vi "createFilePath.vi"(10 "fileSuffix":string, 11 "Base Path":path=path "D:/") -> (2 "appended path":path)   [LabVIEW 2018]
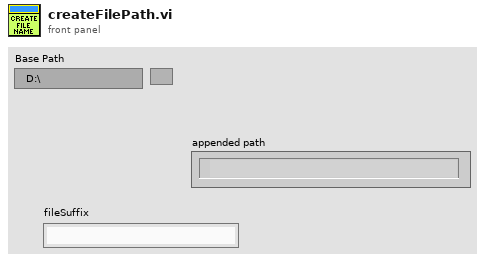
[diagram p1: front panel]
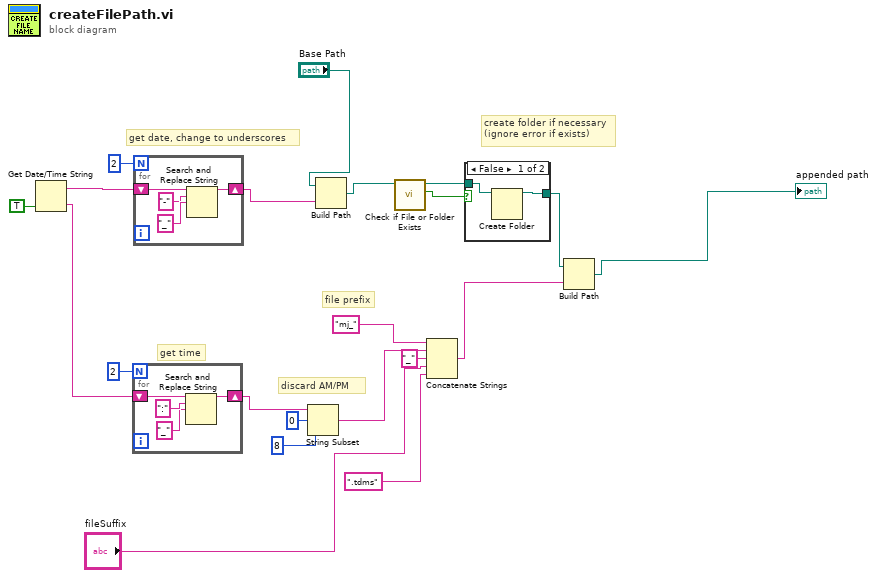
[diagram p0: block diagram]
diagram:
  # "file prefix"
  # "create folder if necessary\n(ignore error if exists)"
  # "get time"
  # "discard AM/PM"
  # "get date, change to underscores"
  n1 = Get Date/Time String(want seconds? (F)=TRUE) -> (date string=w18:string, time string=w17:string)  [unwired: 2 in]
  n2 = for {
    N: 2 -> [_]
    shift-right: [w22] -> w16
    shift-left: w17 -> [w25]
    n3 = Search and Replace String(input string=w25, search string=":", replace string="_" ("replace string (\"\")")) -> (result string=w22:string)  [unwired: 5 in, 3 out]
  }
  n4 = for {
    N: 2 -> [_]
    shift-right: [w26] -> w11
    shift-left: w18 -> [w27]
    n5 = Search and Replace String(input string=w27, search string="-", replace string="_" ("replace string (\"\")")) -> (result string=w26:string)  [unwired: 5 in, 3 out]
  }
  n6 = String Subset(string=w16, offset (0)=0, length (rest)=8 ("length (rest)")) -> (substring=w15:string)
  n7 = Build Path(base path="Base Path", name or relative path=w11) -> (appended path=w7:path)
  n8 = call <vilib>:"Check if File or Folder Exists.vi"("path"=w7) -> ("file or folder exists?"=w6:bool, "dup path"=w5:path)  [unwired: 8 in, 1 out]
  n9 = Concatenate Strings("mj_" ("string"), w15, "_" ("string"), "fileSuffix", ".tdms" ("string")) -> (w9:string)
  n10 = case shown="False" w6 {
    tunnel: [w31 w32] -> w10
    tunnel: w5 -> [w30 w32]
    frame False {
      n11 = Create Folder(path (use dialog)=w30) -> (created path=w31:path)  [unwired: 2 in, 2 out]
    }
    frame True {
    }
  }
  n12 = Build Path(base path=w10, name or relative path=w9) -> (appended path=→"appended path":path)
